vi "Write Actor Core VI Ref.vi"(8 "error in (no error)":errorcluster, 10 "Actor Core VI Ref":refnum<vi>, 11 "AMS Gas Actor in":refnum<class "AMS Gas Actor.lvclass">) -> (0 "error out":errorcluster, 3 "AMS Gas Actor out":refnum<class "AMS Gas Actor.lvclass">)   [LabVIEW 2015, in "AMS UI.lvlib" / "AMS Gas Actor.lvclass"]
uses:
  AMS Gas Actor.lvclass
  AMS Gas Actor.lvclass/AMS Gas Actor.ctl
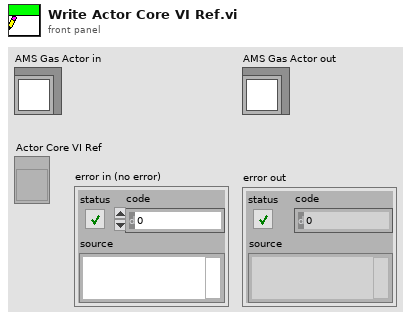
[diagram p1: front panel]
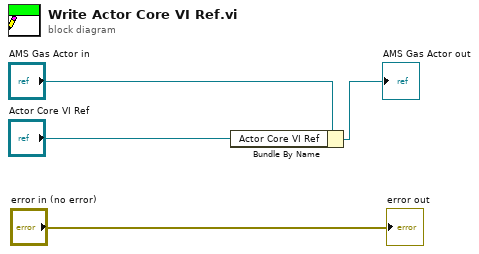
[diagram p0: block diagram]
diagram:
  n1 = Bundle By Name(cluster="AMS Gas Actor in", "Actor Core VI Ref"="Actor Core VI Ref") -> (→"AMS Gas Actor out":refnum<class "AMS Gas Actor.lvclass">)
  "error out" <- "error in (no error)"
